vi "From Variant.vi"(8 "Error In":errorcluster, 10 "Variant":variant, 11 "2D Path In":refnum<class "2D Path.lvclass">) -> (0 "Error Out":errorcluster, 3 "2D Path Out":refnum<class "2D Path.lvclass">)   [LabVIEW 2020, in "NI_VIAnCFGDataStructure.lvlib" / "2D Path.lvclass"]
doc: "Dynamic dispatch interface for conversion of variant LV data to Tree Data classes."
uses:
  <vilib>/addons/analyzer/VIAnCFGDataStructure/Data Types/2D Path/2D Path.lvclass
  <vilib>/addons/analyzer/VIAnCFGDataStructure/Data Types/2D Path/2D Path.lvclass/2D Path.ctl
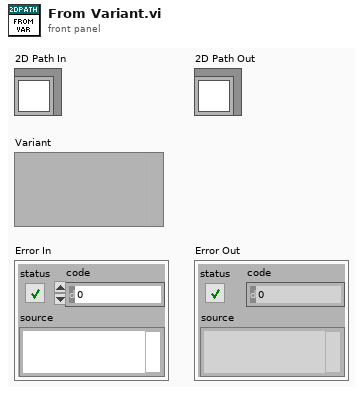
[diagram p1: front panel]
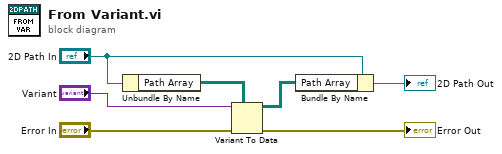
[diagram p0: block diagram]
diagram:
  n1 = Unbundle By Name("2D Path In") -> ("Path Array"=w4:path[][])
  n2 = Variant To Data(error in="Error In", type=w4, Variant="Variant") -> (data=w3:path[][], error out=→"Error Out":errorcluster)
  n3 = Bundle By Name(cluster="2D Path In", "Path Array"=w3) -> (→"2D Path Out":refnum<class "2D Path.lvclass">)
